vi "GetTeamsFromMatch.vi"(10 "Match":string) -> (2 "Teams":string[](array[string]))   [LabVIEW 2017]
uses:
  <vilib>/Utility/config.llb/Read Key (String).vi
  <vilib>/Utility/config.llb/NI_LVConfig.lvlib
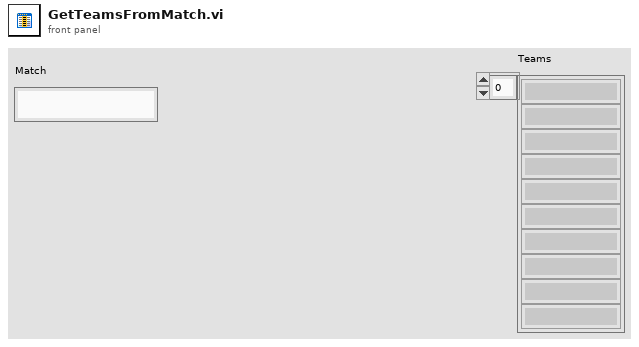
[diagram p1: front panel]
types:
  T1 = typedef "NI_LVConfig.lvlib/Config Data RefNum.ctl" = refnum<k1>
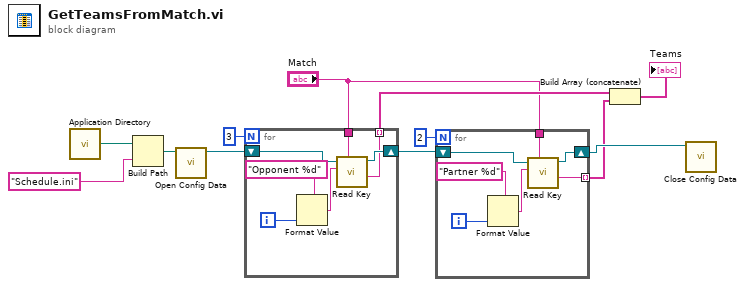
[diagram p0: block diagram]
diagram:
  n1 = call <vilib>:"Application Directory.vi"() -> ("Application Directory"=w4:path)
  n2 = Build Path(base path=w4, name or relative path="Schedule.ini") -> (appended path=w3:path)
  n3 = call <vilib>:"Open Config Data.vi"("configuration file path"=w3) -> ("refnum"=w12:T1)  [unwired: 8 in, 2 out]
  n4 = for {
    N: 3 -> [_]
    tunnel: "Match" -> [w17]
    shift-right: [w16] -> w10
    shift-left: w12 -> [w18]
    tunnel: [w13] -> w6 mode=indexing
    i -> [w14]
    n5 = Format Value(format string="Opponent %d" ("key"), value (0)=w14) -> (output string=w15:string)  [unwired: 1 in]
    n6 = call-poly <vilib>:"Read Key.vi"("section"=w17, "key"=w15, "refnum"=w18) -> ("value"=w13:string, "refnum out"=w16:T1)  [unwired: 5 in, 2 out]
  }
  n7 = for {
    N: 2 -> [_]
    tunnel: "Match" -> [w24]
    shift-right: [w23] -> w8
    shift-left: w10 -> [w25]
    tunnel: [w20] -> w7 mode=indexing
    i -> [w21]
    n8 = Format Value(format string="Partner %d" ("key"), value (0)=w21) -> (output string=w22:string)  [unwired: 1 in]
    n9 = call-poly <vilib>:"Read Key.vi"("section"=w24, "key"=w22, "refnum"=w25) -> ("value"=w20:string, "refnum out"=w23:T1)  [unwired: 5 in, 2 out]
  }
  n10 = Build Array (concatenate)(w6, w7) -> (→"Teams":string[])
  n11 = call <vilib>:"Close Config Data.vi"("refnum"=w8) -> ()  [unwired: 9 in, 2 out]
